vi "Motor_Test.vi"() -> ()   [LabVIEW 2020]
uses:
  <vilib>/DAQmx/write.llb/DAQmx Write (Digital 1D Bool 1Chan 1Samp).vi
  <vilib>/DAQmx/create/channels.llb/DAQmx Create Channel (DO-Digital Output).vi
  <vilib>/DAQmx/miscellaneous.llb/DAQmx Fill In Error Info.vi
panel:
  in  "Delay":i32(knob) scale=20.0..500.0
  in  "Play Button":bool
  out "Coil state":bool[](array[boolean])
  in  "Action":enum16{"Reset", "Set", "Get"}(ring)
  in  "Type":enum16{"Full", "Half", "Torque"}(ring)
  in  "Direction":enum16{"CW", "CCW"}(ring)
  in  "Stop Button":bool
  in  "E stop":bool
  in  "CW":bool
  in  "CCW":bool
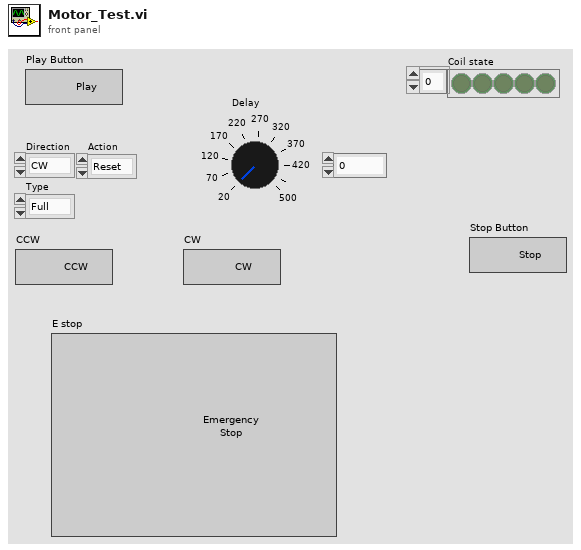
[diagram p1: front panel]
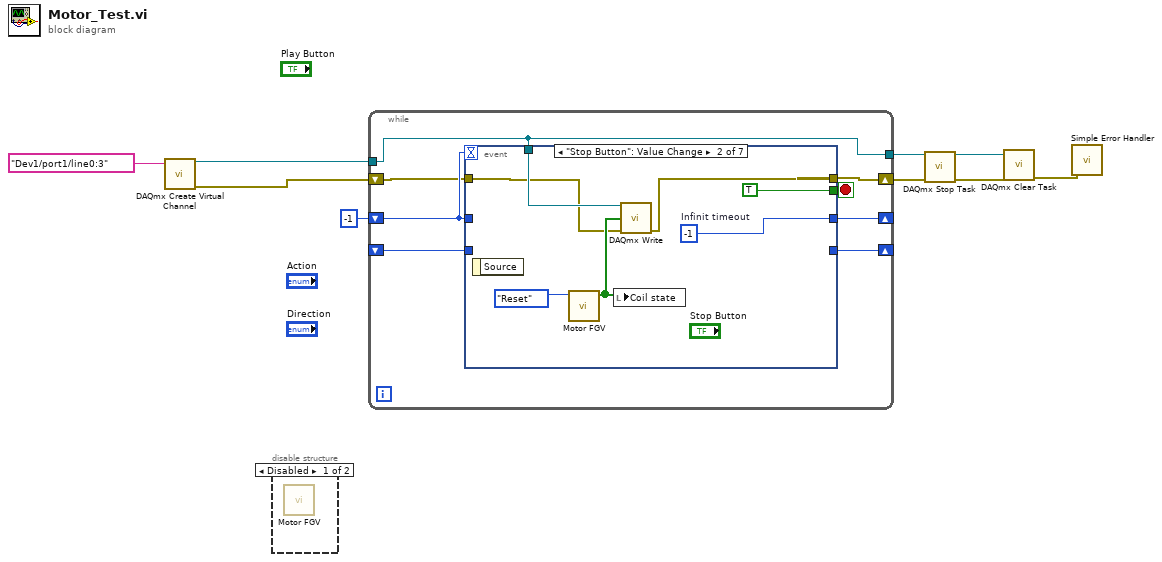
[diagram p0: block diagram]
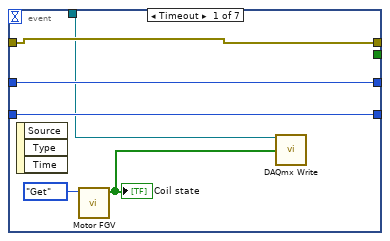
[diagram p3: hidden frame]
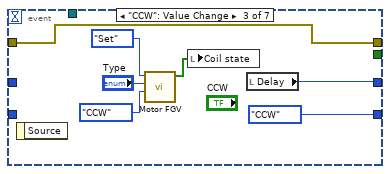
[diagram p4: hidden frame]
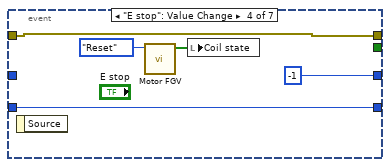
[diagram p5: hidden frame]
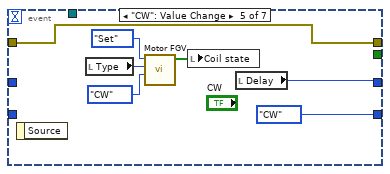
[diagram p6: hidden frame]
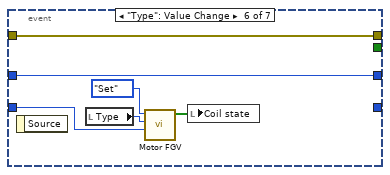
[diagram p7: hidden frame]
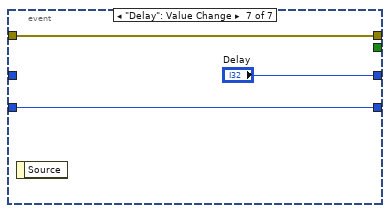
[diagram p8: hidden frame]
diagram:
  n1 = call-poly <vilib>:"DAQmx Create Virtual Channel.vi"("lines"=tag "Dev1/port1/line0:3") -> ("task out"=w7:refnum<k21>, "error out"=w6:errorcluster)  [unwired: 13 in]
  n2 = disable-structure shown="Disabled" {
    frame Disabled {
      n3 = call "Motor FGV.vi"() -> ()  [unwired: 11 in, 1 out]
    }
    frame Enabled {
    }
  }
  n4 = while {
    shift-right: [w15] -> _
    shift-left: -1 -> [w16]
    shift-right: [w14] -> _
    shift-left: _ -> [w13]
    tunnel: w7 -> [w10]
    shift-right: [w11] -> w5
    shift-left: w6 -> [w12]
    tunnel: [w10] -> w2
    stop <- w17 stop-if-true
    n5 = event shown="[1] \"Stop Button\": Value Change" {
      selector: _ -> [_ _ _ _ _ _ _]
      dyn-events: _ -> [_ _ _ _ _ _ _]
      timeout: w16 -> [_ _ _ _ _ _ _]
      tunnel: [_ TRUE _ _ _ _ _] -> w17
      tunnel: w16 -> [w23 _ _ _ _ w55 _]
      tunnel: [w23 w29 w32 -1 ("Infinit timeout") w44 w55 "Delay"] -> w15
      tunnel: [w21 _ enum16{"CW", "CCW"}."CCW" ("Direction") w39 enum16{"CW", "CCW"}."CW" ("Direction") _ w58] -> w14
      tunnel: w13 -> [w21 _ _ w39 _ w53 w58]
      tunnel: [w20 w24 w31 w38 w43 w50 w56] -> w11
      tunnel: w12 -> [w20 w25 w31 w38 w43 w50 w56]
      tunnel: w10 -> [w18 w26 _ _ _ _ _]
      event Timeout {
        n6 = event-data() -> ()  [unwired: 1 in, 3 out]
        n7 = call "Motor FGV.vi"("Action"=enum16{"Reset", "Set", "Get"}."Get") -> ("Coil state"=w19:bool[])  [unwired: 10 in]
        "Coil state" <- w19
        n8 = call-poly <vilib>:"DAQmx Write.vi"("task/channels in"=w18, "data"=w19) -> ()  [unwired: 11 in, 3 out]
      }
      event "Stop Button": Value Change {
        w29 = -1  # Infinit timeout
        n9 = event-data() -> ()  [unwired: 1 in, 1 out]
        n10 = call "Motor FGV.vi"("Action"=enum16{"Reset", "Set", "Get"}."Reset") -> ("Coil state"=w27:bool[])  [unwired: 10 in]
        n11 = local write "Coil state"(w27) -> ()
        n12 = call-poly <vilib>:"DAQmx Write.vi"("task/channels in"=w26, "data"=w27, "error in"=w25) -> ("error out"=w24:errorcluster)  [unwired: 10 in, 2 out]
      }
      event "CCW": Value Change {
        n13 = event-data() -> ()  [unwired: 1 in, 1 out]
        n14 = call "Motor FGV.vi"("Direction"=enum16{"CW", "CCW"}."CCW", "Type"="Type", "Action"=enum16{"Reset", "Set", "Get"}."Set") -> ("Coil state"=w34:bool[])  [unwired: 8 in]
        n15 = local write "Coil state"(w34) -> ()
        n16 = local read "Delay"() -> (w32:i32)
      }
      event "E stop": Value Change {
        n17 = event-data() -> ()  [unwired: 1 in, 1 out]
        n18 = call "Motor FGV.vi"("Action"=enum16{"Reset", "Set", "Get"}."Reset") -> ("Coil state"=w41:bool[])  [unwired: 10 in]
        n19 = local write "Coil state"(w41) -> ()
      }
      event "CW": Value Change {
        n20 = event-data() -> ()  [unwired: 1 in, 1 out]
        n21 = local read "Type"() -> (w46:enum16{"Full", "Half", "Torque"})
        n22 = call "Motor FGV.vi"("Direction"=enum16{"CW", "CCW"}."CW", "Type"=w46, "Action"=enum16{"Reset", "Set", "Get"}."Set") -> ("Coil state"=w47:bool[])  [unwired: 8 in]
        n23 = local write "Coil state"(w47) -> ()
        n24 = local read "Delay"() -> (w44:i32)
      }
      event "Type": Value Change {
        n25 = event-data() -> ()  [unwired: 1 in, 1 out]
        n26 = local read "Type"() -> (w52:enum16{"Full", "Half", "Torque"})
        n27 = call "Motor FGV.vi"("Direction"=w53, "Type"=w52, "Action"=enum16{"Reset", "Set", "Get"}."Set") -> ("Coil state"=w51:bool[])  [unwired: 8 in]
        n28 = local write "Coil state"(w51) -> ()
      }
      event "Delay": Value Change {
        n29 = event-data() -> ()  [unwired: 1 in, 1 out]
      }
    }
  }
  n30 = call <vilib>:"DAQmx Stop Task.vi"("task/channels in"=w2, "error in"=w5) -> ("task out"=w1:refnum<k21>, "error out"=w4:errorcluster)  [unwired: 12 in]
  n31 = call <vilib>:"DAQmx Clear Task.vi"("task in"=w1, "error in"=w4) -> ("error out"=w3:errorcluster)  [unwired: 13 in]
  n32 = call <vilib>:"Simple Error Handler.vi"("error in (no error)"=w3) -> ()  [unwired: 4 in, 5 out]
